vi "Segmentacion.vi"(0 "R":u8=160, 1 "UR":u8, 2 "G":u8=160, 3 "UG":u8, 4 "B":u8=160, 5 "UB":u8, 7 "TR":u8=10, 9 "TG":u8=10, 11 "TB":u8=10) -> (14 "ColorSegmentado":u32(colorbox), 19 "binario":bool)   [LabVIEW 2021]
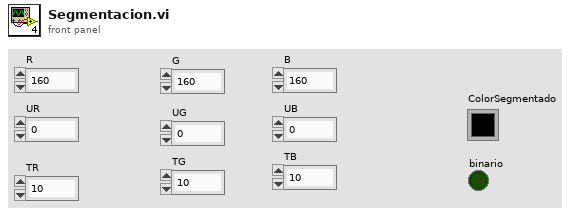
[diagram p1: front panel]
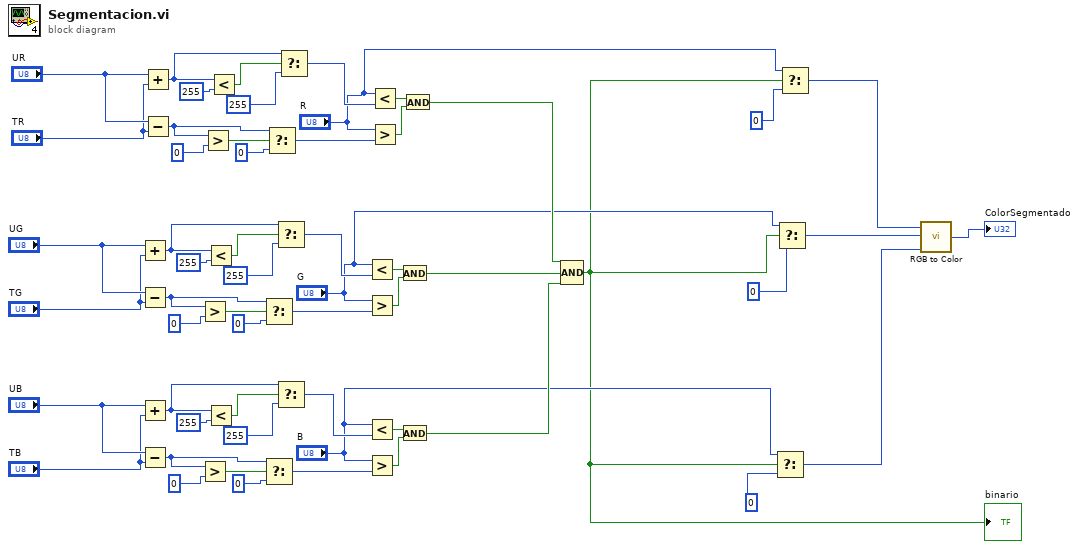
[diagram p0: block diagram]
diagram:
  n1 = Add(x="UG", y="TG") -> (x+y=w41:u8)
  n2 = Subtract(x="UG", y="TG") -> (x-y=w45:u8)
  n3 = Add(x="UB", y="TB") -> (x+y=w13:u8)
  n4 = Subtract(x="UB", y="TB") -> (x-y=w17:u8)
  n5 = Add(x="UR", y="TR") -> (x+y=w27:u8)
  n6 = Subtract(x="UR", y="TR") -> (x-y=w31:u8)
  n7 = Greater?(x=w45, y=u8 0) -> (0:w47:bool)
  n8 = Greater?(x=w17, y=u8 0) -> (0:w19:bool)
  n9 = Greater?(x=w31, y=u8 0) -> (0:w33:bool)
  n10 = Less?(x=w41, y=u8 255) -> (x < y?=w42:bool)
  n11 = Less?(x=w13, y=u8 255) -> (x < y?=w14:bool)
  n12 = Less?(x=w27, y=u8 255) -> (x < y?=w28:bool)
  n13 = Select(t=w45, s=w47, f=u8 0) -> (s? t:f=w44:u8)
  n14 = Select(t=w17, s=w19, f=u8 0) -> (s? t:f=w16:u8)
  n15 = Select(t=w31, s=w33, f=u8 0) -> (s? t:f=w30:u8)
  n16 = Select(t=w41, s=w42, f=u8 255) -> (s? t:f=w39:u8)
  n17 = Select(t=w13, s=w14, f=u8 255) -> (s? t:f=w11:u8)
  n18 = Select(t=w27, s=w28, f=u8 255) -> (s? t:f=w25:u8)
  n19 = Less?(x="G", y=w39) -> (x < y?=w54:bool)
  n20 = Greater?(x="G", y=w44) -> (0:w53:bool)
  n21 = Less?(x="B", y=w11) -> (x < y?=w24:bool)
  n22 = Greater?(x="B", y=w16) -> (0:w23:bool)
  n23 = Less?(x="R", y=w25) -> (x < y?=w38:bool)
  n24 = Greater?(x="R", y=w30) -> (0:w37:bool)
  n25 = And(x=w54, y=w53) -> (x .and. y?=w9:bool)
  n26 = And(x=w24, y=w23) -> (x .and. y?=w10:bool)
  n27 = And(x=w38, y=w37) -> (x .and. y?=w8:bool)
  n28 = Compound Arithmetic op=AND(w8, w9, w10) -> (w1:bool)
  "binario" <- w1
  n29 = Select(t="B", s=w1, f=u8 0) -> (s? t:f=w2:u8)
  n30 = Select(t="G", s=w1, f=u8 0) -> (s? t:f=w3:u8)
  n31 = Select(t="R", s=w1, f=u8 0) -> (s? t:f=w4:u8)
  n32 = call <vilib>:"RGB to Color.vi"("B"=w2, "G"=w3, "R"=w4) -> ("Color"=→"ColorSegmentado":u32)
